vi "Pockels Cal-Check meas AI exists.vi"(8 "error in (no error)":errorcluster) -> (0 "error out":errorcluster, 2 "Power-meter meas. AI channel exists":bool, 3 "Power meter AI (dupl)":tag)   [LabVIEW 2017]
uses:
  Globals/gl_Calibration globals.vi
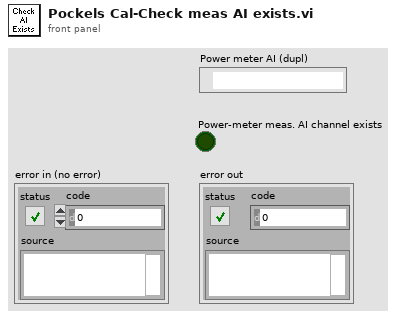
[diagram p1: front panel]
types:
  T1 = enum16{"AI.PhysicalChans", "AO.PhysicalChans", "DI.Ports", "DO.Ports", "CtrIn.PhysicalChans", "CtrOut.PhysicalChans"}
  T2 = typedef "Pre-AOL Z wizard refs.ctl" = cluster{"VI's reference":refnum<vi>, "Calibration Mode":refnum<vi>, "Cal points":refnum<vi>, "Channel Selector":refnum<vi>, "Message":refnum<vi>, "Back":refnum<vi>, "Next":refnum<vi>, "Power meter AI":refnum<vi>, "2D Picture":refnum<vi>, "Note":refnum<vi>}
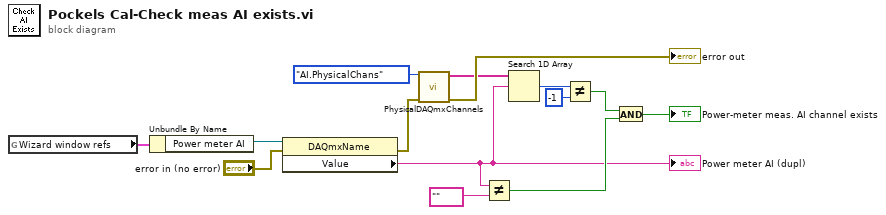
[diagram p0: block diagram]
diagram:
  n1 = global read "gl_Calibration globals.vi" "Wizard window refs"() -> (w4:T2)
  n2 = Unbundle By Name(w4) -> ("Power meter AI"=w5:refnum<vi>)
  n3 = property on="Property Node" class="DAQmxName"(reference=w5, error in="error in (no error)") -> (error out=w1:errorcluster, "Value"=w3:string)  [unwired: 1 out]
  "Power meter AI (dupl)" <- w3
  n4 = call "PhysicalDAQmxChannels.vi"("error in (no error)"=w1, "Channel type"=T1."AI.PhysicalChans") -> ("error out"=→"error out":errorcluster, "Channels of elected type"=w8:tag[])  [unwired: 8 in]
  n5 = Not Equal?(x=w3, y=tag "" ("Power meter AI")) -> (x != y?=w12:bool)
  n6 = Search 1D Array(1D array=w8, element=w3) -> (index of element=w9:i32)  [unwired: 1 in]
  n7 = Not Equal?(x=w9, y=-1) -> (x != y?=w11:bool)
  n8 = And(x=w11, y=w12) -> (x .and. y?=→"Power-meter meas. AI channel exists":bool)
